vi "Config Waitfor Trgmode.vi"(8 "error in":errorcluster, 10 "Trigger Mode (Buffer)":u16(ring) items=["Buffer", "Give_Err"], 11 "VISA resource name":refnum<visa-resource-name>) -> (0 "error out":errorcluster, 3 "VISA resource name out":refnum<visa-resource-name>)   [LabVIEW 2019, in "Andeen-Hagerling 2700(400 firmware).lvlib"]
doc: "This command determines what happens to external trigger pulses that arrive when no command has been executed to receive them."
uses:
  Andeen-Hagerling 2700(400 firmware).lvlib
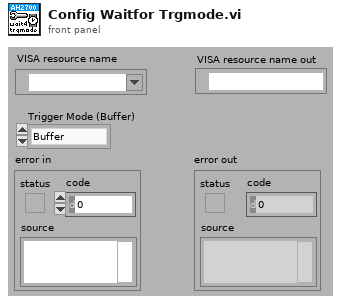
[diagram p1: front panel]
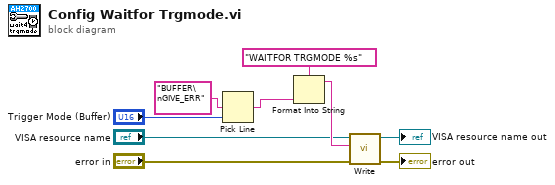
[diagram p0: block diagram]
diagram:
  n1 = Pick Line(multi-line string="BUFFER\nGIVE_ERR", line index="Trigger Mode (Buffer)") -> (output string=w1:string)  [unwired: 1 in]
  n2 = Format Into String(format string="WAITFOR TRGMODE %s", w1) -> (resulting string=w6:string)  [unwired: 2 in, 1 out]
  n3 = call "Write.vi"("error in"="error in", "command"=w6, "VISA resource name"="VISA resource name") -> ("error out"=→"error out":errorcluster, "VISA resource name out"=→"VISA resource name out":refnum<visa-resource-name>)  [unwired: 7 in]
